vi "LaserCal-Initialize (PT).vi"(0 "Settings":T1={"System ID"={"Name"="", "Laser SN"="", "Wavelength (nm)"=0.0, "Fiber diameter (um)"=0.0, "Power setting"=0.0}, "Sensor"={"Average (ms)"=0.0, "Range"=""}, "Meter"={"Vcommand"=0.0, "scale"=enum."linear", "Pulsed"=FALSE, "Pulse width (ms)"=0.0, "Pulse rate (Hz)"=0.0, "mode"=enum."Voltage only"}, "Static"={"Stimulus"={"scale"=enum."linear", "Voltage"=""}, "Response"={"Settle time (s)"=1.0, "Tmeasure (s)"=2.0}}, "Pulsed"={"Stimulus"={"Vcommand Expr"="", "Width Expr"="", "mode"=enum."Voltage only", "Rate Expr"="", "randomize"=FALSE}, "Response"={"Settle time (s)"=1.0, "Tmeasure (s)"=2.0, "Repeats"=10}}, "Options"={"current"=FALSE, "save current"=FALSE, "mA/V"=0.0}}, 11 "error in (no error)":errorcluster) -> (2 "Taverage (ms)":dbl, 4 "Stimulus out":T3, 6 "Runtime State":T12={"AO Channels"=[], "Fs (Hz)"=100000.0, "Npts"=1, "conversion"=0.0}, 8 "SCL":T10[](array[typedef]), 10 "First SCL Element":T10, 14 "I-O Data":T11, 15 "error out":errorcluster)   [LabVIEW 2015]
uses:
  Typedefs/LaserCal-Meter Stimulus.ctl
  Typedefs/LaserCal-Control Mode.ctl
  Typedefs/LaserCal-Meter Runtime State.ctl
  Typedefs/LaserCal-Data (PT).ctl
  Typedefs/LaserCal-StimConList Element.ctl
  Typedefs/LaserCal-Settings.ctl
  Typedefs/LaserCal-System ID.ctl
  Typedefs/LaserCal-IO Stimulus Params.ctl
  Typedefs/LaserCal-IO Response Params.ctl
  Typedefs/LaserCal-Stimulus Params.ctl
  Typedefs/LaserCal-Response (PT).ctl
  Typedefs/LaserCal-Options.ctl
panel:
  in  "Fs (Hz)":dbl=100000.0
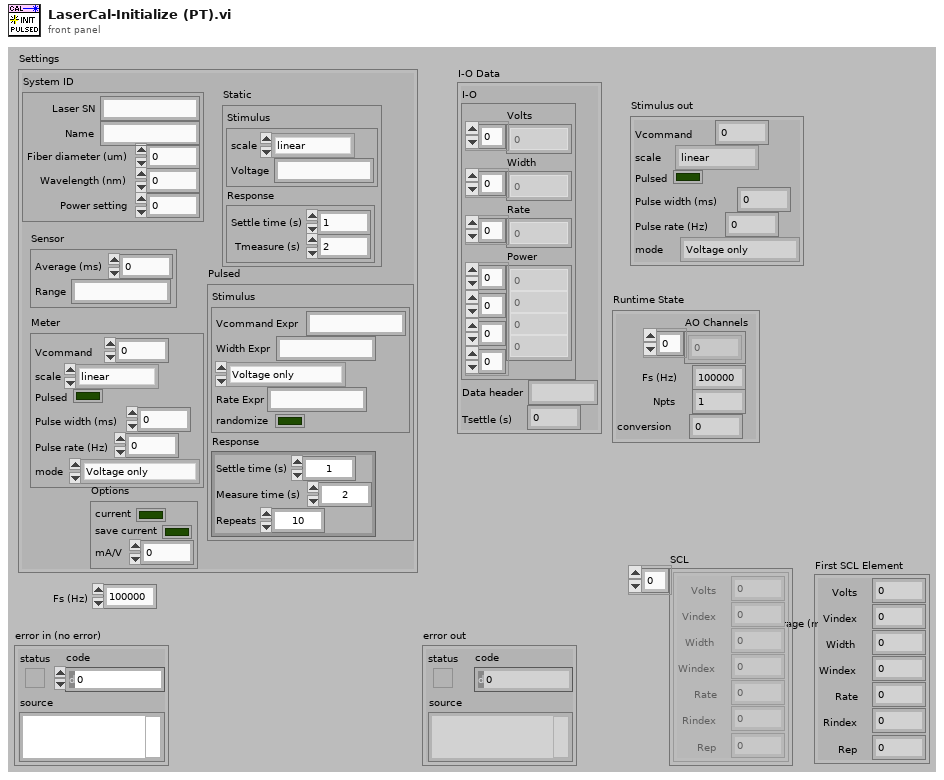
[diagram p1: front panel]
types:
  T1 = typedef "LaserCal-Settings.ctl" = cluster{"System ID":T2, "Sensor":cluster{"Average (ms)":dbl, "Range":string}, "Meter":T3, "Static":cluster{"Stimulus":T5, "Response":T6}, "Pulsed":cluster{"Stimulus":T7, "Response":T8}, "Options":T9}
  T2 = typedef "LaserCal-System ID.ctl" = cluster{"Name":string, "Laser SN":string, "Wavelength (nm)":dbl, "Fiber diameter (um)":dbl, "Power setting":dbl}
  T3 = typedef "LaserCal-Meter Stimulus.ctl" = cluster{"Vcommand":dbl, "scale":enum16{"linear", "dB"}, "Pulsed":bool, "Pulse width (ms)":dbl, "Pulse rate (Hz)":dbl, "mode":T4}
  T4 = typedef "LaserCal-Control Mode.ctl" = enum16{"Voltage only", "Voltage + Enable"}
  T5 = typedef "LaserCal-IO Stimulus Params.ctl" = cluster{"scale":enum16{"linear", "dB"}, "Voltage":string}
  T6 = typedef "LaserCal-IO Response Params.ctl" = cluster{"Settle time (s)":dbl, "Tmeasure (s)":dbl}
  T7 = typedef "LaserCal-Stimulus Params.ctl" = cluster{"Vcommand Expr":string, "Width Expr":string, "mode":T4, "Rate Expr":string, "randomize":bool}
  T8 = typedef "LaserCal-Response (PT).ctl" = cluster{"Settle time (s)":dbl, "Tmeasure (s)":dbl, "Repeats":i32}
  T9 = typedef "LaserCal-Options.ctl" = cluster{"current":bool, "save current":bool, "mA/V":dbl}
  T10 = typedef "LaserCal-StimConList Element.ctl" = cluster{"Volts":dbl, "Vindex":i32, "Width":dbl, "Windex":i32, "Rate":dbl, "Rindex":i32, "Rep":i32}
  T11 = typedef "LaserCal-Data (PT).ctl" = cluster{"I-O":cluster{"Volts":dbl[], "Width":dbl[], "Rate":dbl[], "Power":dbl[][][][]}, "Data header":string, "Tsettle (s)":dbl}
  T12 = typedef "LaserCal-Meter Runtime State.ctl" = cluster{"AO Channels":i32[], "Fs (Hz)":dbl, "Npts":i32, "conversion":dbl}
  T13 = cluster{"Array":dbl[], "Array":dbl[], "Array":dbl[], dbl[][][][]}
  T14 = cluster{cluster{"Array":dbl[], "Array":dbl[], "Array":dbl[], dbl[][][][]}, "Header out":string, "Settle time (s)":dbl}
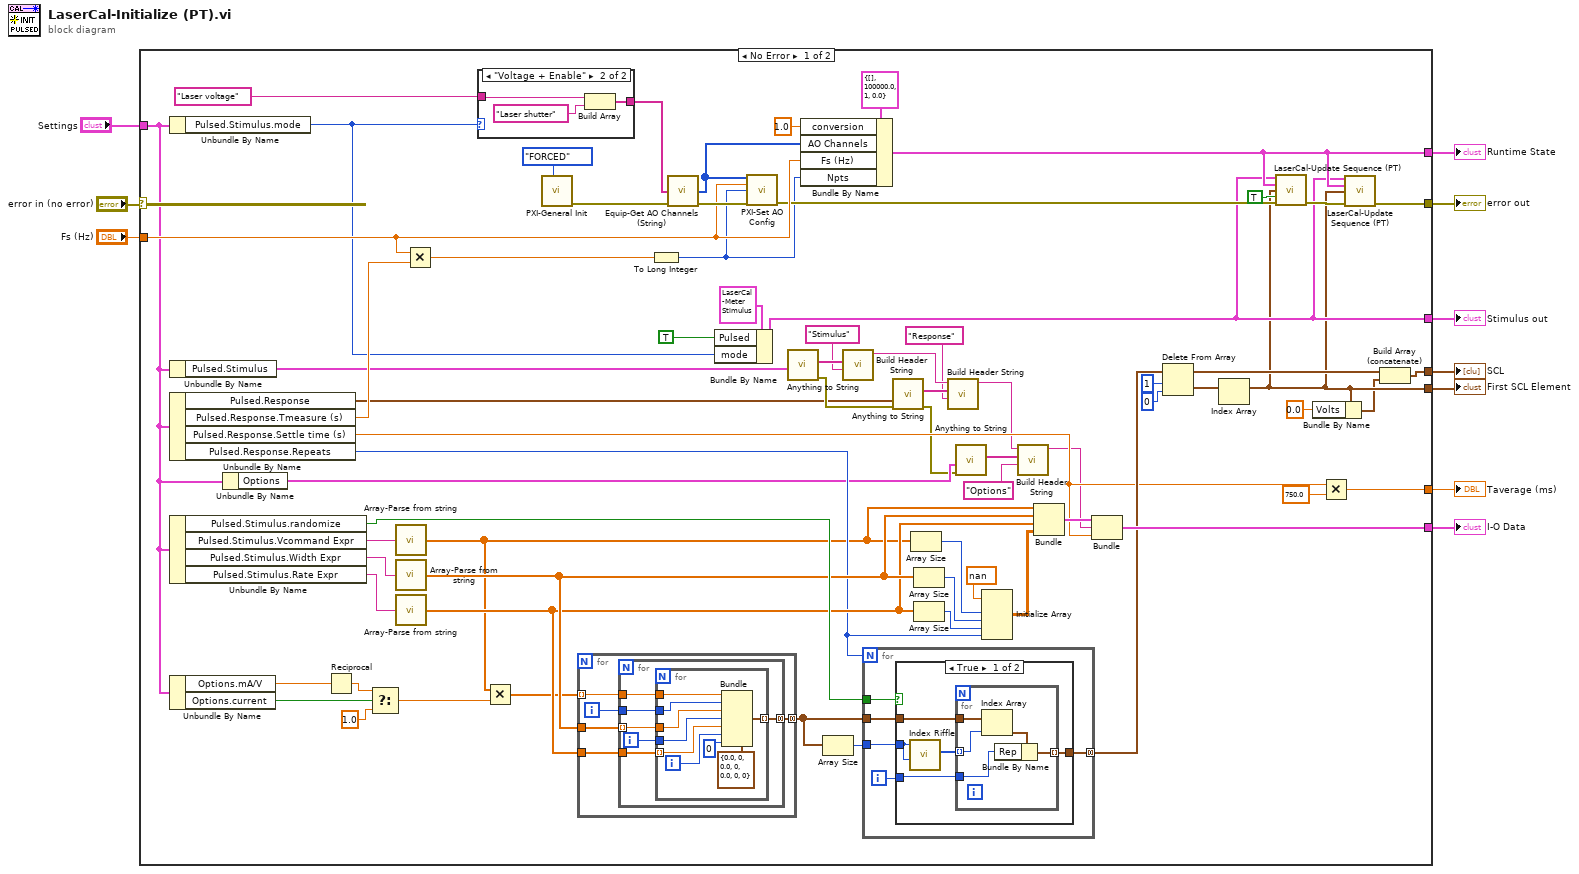
[diagram p0: block diagram]
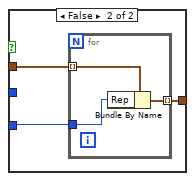
[diagram p2: hidden frame]
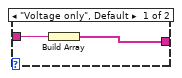
[diagram p3: hidden frame]
diagram:
  n1 = case shown="No Error" "error in (no error)" {
    selector: "error in (no error)" -> [_ w128]
    tunnel: [w72 w128] -> w9
    tunnel: "Fs (Hz)" -> [w76 _]
    tunnel: [w44 _] -> w7
    tunnel: [w73 _] -> w4
    tunnel: [w43 _] -> w6
    tunnel: "Settings" -> [w20 _]
    tunnel: [w37 _] -> w5
    tunnel: [w35 _] -> w3
    tunnel: [w39 _] -> w2
    frame No Error {
      n2 = Unbundle By Name(w20) -> ("Pulsed.Stimulus.mode"=w31:T4)
      n3 = Unbundle By Name(w20) -> ("Pulsed.Stimulus"=w23:T7)
      n4 = Unbundle By Name(w20) -> ("Pulsed.Response"=w24:T8, "Pulsed.Response.Tmeasure (s)"=w66:dbl, "Pulsed.Response.Settle time (s)"=w45:dbl, "Pulsed.Response.Repeats"=w48:i32)
      n5 = Unbundle By Name(w20) -> ("Pulsed.Stimulus.randomize"=w56:bool, "Pulsed.Stimulus.Vcommand Expr"=w61:string, "Pulsed.Stimulus.Width Expr"=w60:string, "Pulsed.Stimulus.Rate Expr"=w59:string)
      n6 = Unbundle By Name(w20) -> ("Options.mA/V"=w28:dbl, "Options.current"=w29:bool)
      n7 = Unbundle By Name(w20) -> ("Options"=w19:T9)
      n8 = Reciprocal(x=w28) -> (1/x=w27:dbl)
      n9 = Select(t=w27, s=w29, f=1.0) -> (s? t:f=w25:dbl)
      n10 = call "Array-Parse from string.vi"("String"=w61) -> ("Array"=w22:dbl[])  [unwired: 13 in, 1 out]
      n11 = call "Array-Parse from string.vi"("String"=w60) -> ("Array"=w50:dbl[])  [unwired: 13 in, 1 out]
      n12 = call "Array-Parse from string.vi"("String"=w59) -> ("Array"=w49:dbl[])  [unwired: 13 in, 1 out]
      n13 = Multiply(x=w76, y=w66) -> (x*y=w65:dbl)
      n14 = case shown="\"Voltage + Enable\"" w31 {
        tunnel: "Laser voltage" ("String") -> [w124 w127]
        tunnel: [w123 w125] -> w68
        frame "Voltage only", Default {
          n15 = Build Array(w124) -> (w123:string[])
        }
        frame "Voltage + Enable" {
          n16 = Build Array(w127, "Laser shutter" ("String")) -> (w125:string[])
        }
      }
      n17 = Multiply(x=w22, y=w25) -> (x*y=w21:dbl[])
      n18 = call "PXI-General Init.vi"("Double Buffer Mode"=enum32{"OFF", "ENABLED", "FORCED"}."FORCED") -> ("error out"=w80:errorcluster)  [unwired: 10 in]
      n19 = for {
        tunnel: w21 -> [w105] mode=indexing
        tunnel: w50 -> [w107]
        tunnel: w49 -> [w106]
        tunnel: [w103] -> w58 mode=concatenating
        i -> [w104]
        n20 = for {
          tunnel: w107 -> [w111] mode=indexing
          tunnel: w106 -> [w113]
          tunnel: w105 -> [w112]
          tunnel: w104 -> [w110]
          tunnel: [w108] -> w103 mode=concatenating
          i -> [w109]
          n21 = for {
            tunnel: w113 -> [w118] mode=indexing
            tunnel: w112 -> [w122]
            tunnel: w111 -> [w120]
            tunnel: w110 -> [w121]
            tunnel: w109 -> [w119]
            tunnel: [w115] -> w108 mode=indexing
            i -> [w117]
            n22 = Bundle(cluster=T10 {"Volts"=0.0, "Vindex"=0, "Width"=0.0, "Windex"=0, "Rate"=0.0, "Rindex"=0, "Rep"=0} ("SCL Element"), "Volts"=w122, "Vindex"=w121, "Width"=w120, "Windex"=w119, "Rate"=w118, "Rindex"=w117, "Rep"=0) -> (w115:T10)
          }
        }
      }
      n23 = To Long Integer(number=w65) -> (32bit integer=w67:i32)
      n24 = call "Equip-Get AO Channels (String).vi"("Channel Names"=w68, "error in (no error)"=w80) -> ("AO Channels"=w77:i32[], "error out"=w79:errorcluster)  [unwired: 12 in]
      n25 = Bundle By Name(cluster=T3 {"Vcommand"=0.0, "scale"=enum."linear", "Pulsed"=FALSE, "Pulse width (ms)"=0.0, "Pulse rate (Hz)"=0.0, "mode"=enum."Voltage only"} ("Stimulus"), "Pulsed"=TRUE, "mode"=w31) -> (w43:T3)
      n26 = call "PXI-Set AO Config.vi"("AO Channels"=w77, "Sampling Rate (Hz)"=w76, "Buffer Size"=w67, "error in (no error)"=w79) -> ("error out"=w71:errorcluster)  [unwired: 11 in]
      n27 = call "Anything to String.vi"("Anything"=w23) -> ("Error Out"=w62:errorcluster, "Strings[]"=w64:string[])  [unwired: 8 in, 1 out]
      n28 = Bundle By Name(cluster=T12 {"AO Channels"=[], "Fs (Hz)"=100000.0, "Npts"=1, "conversion"=0.0} ("Runtime State"), "conversion"=1.0, "AO Channels"=w77, "Fs (Hz)"=w76, "Npts"=w67) -> (w44:T12)
      n29 = Array Size(array=w58) -> (size(s)=w57:i32)
      n30 = call "Build Header String.vi"("Section"="Stimulus", "Strings[]"=w64) -> ("Header out"=w63:string)  [unwired: 9 in]
      n31 = for {
        N: w48 -> [_]
        tunnel: w58 -> [w85]
        tunnel: w57 -> [w86]
        tunnel: [w83] -> w54 mode=concatenating
        tunnel: w56 -> [w82]
        i -> [w84]
        n32 = case shown="True" w82 {
          tunnel: w86 -> [w91 _]
          tunnel: w85 -> [w89 w99]
          tunnel: w84 -> [w88 w98]
          tunnel: [w87 w97] -> w83
          frame True {
            n33 = call "Index Riffle.vi"("NRiffle"=w91, "N"=w91) -> ("Riffled Indices"=w90:i32[])  [unwired: 9 in]
            n34 = for {
              tunnel: w90 -> [w95] mode=indexing
              tunnel: w89 -> [w96]
              tunnel: w88 -> [w93]
              tunnel: [w92] -> w87 mode=indexing
              n35 = Index Array(array=w96, index=w95) -> (element=w94:T10)
              n36 = Bundle By Name(cluster=w94, "Rep"=w93) -> (w92:T10)
            }
          }
          frame False {
            n37 = for {
              tunnel: w99 -> [w100] mode=indexing
              tunnel: w98 -> [w102]
              tunnel: [w101] -> w97 mode=indexing
              n38 = Bundle By Name(cluster=w100, "Rep"=w102) -> (w101:T10)
            }
          }
        }
      }
      n39 = call "Anything to String.vi"("Error In"=w62, "Anything"=w24) -> ("Error Out"=w18:errorcluster, "Strings[]"=w70:string[])  [unwired: 7 in, 1 out]
      n40 = Array Size(array=w22) -> (size(s)=w74:i32)
      n41 = Array Size(array=w50) -> (size(s)=w52:i32)
      n42 = Array Size(array=w49) -> (size(s)=w51:i32)
      n43 = call "Build Header String.vi"("Section"="Response", "Strings[]"=w70, "Header in"=w63) -> ("Header out"=w17:string)  [unwired: 8 in]
      n44 = call "Anything to String.vi"("Error In"=w18, "Anything"=w19) -> ("Strings[]"=w15:string[])  [unwired: 7 in, 2 out]
      n45 = Initialize Array(nan ("element"), w74, w52, w51, w48) -> (w55:dbl[][][][])
      n46 = call "Build Header String.vi"("Section"="Options", "Strings[]"=w15, "Header in"=w17) -> ("Header out"=w16:string)  [unwired: 8 in]
      n47 = Bundle("Array"=w22, "Array"=w50, "Array"=w49, w55) -> (w53:T13)  [unwired: 1 in]
      n48 = Bundle(w53, "Header out"=w16, "Settle time (s)"=w45) -> (w73:T14)  [unwired: 1 in]
      n49 = Delete From Array(array=w54, length=1, index=0) -> (deleted portion=w41:T10[], array with subset deleted=w40:T10[])
      n50 = Index Array(array=w41) -> (element=w39:T10)  [unwired: 1 in]
      n51 = call "LaserCal-Update Sequence (PT).vi"("Stimulus (I-O)"=w43, "Runtime State"=w44, "SCL Element"=w39, "Start?"=TRUE, "error in (no error)"=w71) -> ("error out"=w47:errorcluster)  [unwired: 10 in]
      n52 = Bundle By Name(cluster=w39, "Volts"=0.0) -> (w36:T10)
      n53 = Multiply(x=w45, y=750.0) -> (x*y=w35:dbl)
      n54 = call "LaserCal-Update Sequence (PT).vi"("Stimulus (I-O)"=w43, "Runtime State"=w44, "SCL Element"=w39, "error in (no error)"=w47) -> ("error out"=w72:errorcluster)  [unwired: 11 in]
      n55 = Build Array (concatenate)(w40, w36) -> (w37:T10[])
    }
    frame Error {
    }
  }
  "error out" <- w9
  "Stimulus out" <- w6
  "Runtime State" <- w7
  "Taverage (ms)" <- w3
  "I-O Data" <- w4
  "SCL" <- w5
  "First SCL Element" <- w2
